vi "hw7p6_hickey (1).vi"() -> ()   [LabVIEW 2014]
uses:
  <vilib>/MakerHub/LINX/Private/Type Defs/User Platform.ctl
  <vilib>/MakerHub/LINX/Private/Type Defs/Interface.ctl
  <vilib>/MakerHub/LINX/Public/Peripherals/Digital/Digital Write 1 Chan.vi
  <vilib>/MakerHub/LINX/LMH-LINX.lvlib
panel:
  out "Error Out 2":errorcluster
  in  "milliseconds to wait":u32
  in  "DO Channel":u8
  out "Error Out":errorcluster
  in  "Serial Port":refnum<visa-resource-name>="N/A"
  in  "Interface":T1
  in  "Platform":T2
  in  "stop":bool
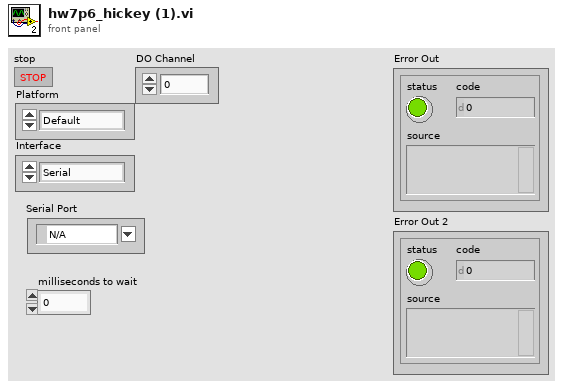
[diagram p1: front panel]
types:
  T1 = typedef "LMH-LINX.lvlib/Interface.ctl" = enum16{"Serial", "TCP"}
  T2 = typedef "LMH-LINX.lvlib/User Platform.ctl" = enum16{"Default", "LINX", "myRIO"}
  T3 = typedef "LMH-LINX.lvlib/LINX Ref.ctl" = cluster{"Platform":T4, "Interface":T1, "LINX Device Config":T5}
  T4 = typedef "LMH-LINX.lvlib/Platform.ctl" = enum16{"LINX", "myRIO"}
  T5 = typedef "LMH-LINX.lvlib/Device.lvlib/LINX Device Config.ctl" = cluster{"Interface":T1, "COM Port":refnum<visa-resource-name>, "TCP Configuration":T6, "Device Family":u8, "Device ID":u8, "Device Name":string, "TCP Ref":refnum<k5>, "Channels":T7}
  T6 = typedef "LMH-LINX.lvlib/Device.lvlib/TCP Config.ctl" = cluster{"IP Address":string, "Port":u16}
  T7 = typedef "LMH-LINX.lvlib/Channels.ctl" = cluster{"DI":u8[], "DO":u8[], "AI":u8[], "AO":u8[], "PWM":u8[], "QE":u8[], "UART":u8[], "I2C 2":u8[], "SPI":u8[], "CAN":u8[], "Servo":u8[], "AI Ref (V)":dbl, "AO Ref (V)":dbl, "AO Resolution (Bits)":u8}
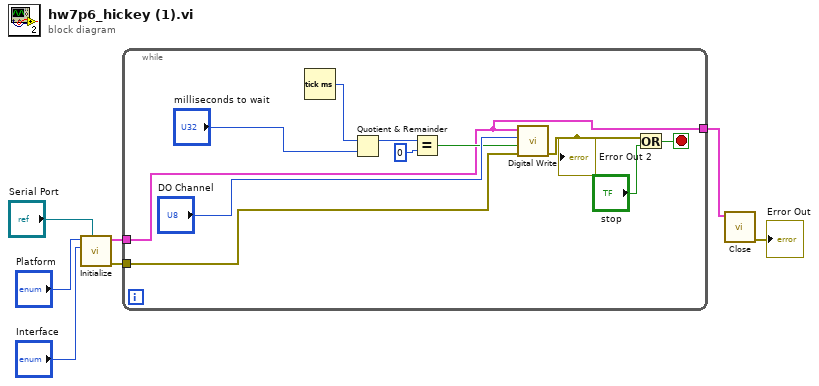
[diagram p0: block diagram]
diagram:
  n1 = call <vilib>:"Initialize.vi"("Serial Port"="Serial Port", "Interface"="Interface", "Platform"="Platform") -> ("Error Out"=w4:errorcluster, "LINX Ref"=w2:T3)  [unwired: 6 in, 1 out]
  n2 = while {
    tunnel: w4 -> [w11]
    tunnel: w2 -> [w8]
    tunnel: [w8] -> w1
    stop <- w17 stop-if-true
    n3 = Tick Count (ms)() -> (millisecond timer value=w16:u32)
    n4 = Quotient & Remainder(x=w16, y="milliseconds to wait") -> (x-y*floor(x/y)=w14:u32)  [unwired: 1 out]
    n5 = Equal?(x=w14, y=u32 0) -> (x = y?=w10:bool)
    n6 = call-poly <vilib>:"Digital Write.vi"("Error In"=w11, "Output Value"=w10, "DO Channel"="DO Channel", "LINX Resource"=w8) -> ("Error Out"=w9:errorcluster)  [unwired: 6 in, 1 out]
    "Error Out 2" <- w9
    n7 = Or(x=w9, y="stop") -> (x .or. y?=w17:bool)
  }
  n8 = call <vilib>:"Close.vi"("LINX Resource"=w1) -> ("Error Out"=→"Error Out":errorcluster)  [unwired: 9 in, 1 out]
